vi "CFTS-Parse Data Header.vi"(8 "error in (no error)":errorcluster, 10 "Header string":string, 11 "Cluster Ref In":refnum<vi>) -> (0 "error out":errorcluster, 3 "Cluster Ref Out":refnum<vi>)   [LabVIEW 2020]
uses:
  <vilib>/regexp/Match Regular Expression.xnode
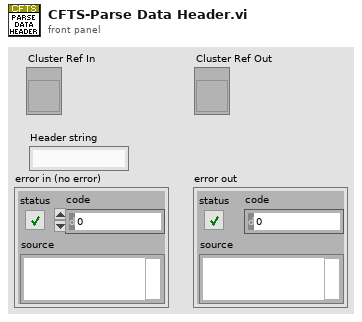
[diagram p1: front panel]
types:
  T1 = typedef "VariantType.lvlib/Type.ctl" = enum8{"Invalid Type", "Void", "I8", "I16", "I32", "I64", "U8", "U16", "U32", "U64", "Single Float", "Double Float", "Extended Float", "Single Complex", "Double Complex", "Extended Complex", "Enum U8", "Enum U16", "Enum U32", "Enum U64", "Single Float With Unit", "Double Float With Unit", "Extended Float With Unit", "Single Complex with Unit", "Double Complex with Unit", "Extended Complex with Unit", "Boolean", "String", "Path", "Picture", "Tag", "Array", "Cluster", "Variant", "LV Variant", "Waveform", "Timestamp", "Digital Waveform", "Digital Data", "ExpressData", "Refnum", "External Data", "VI", "Poly VI", "LabVIEW Class Instance", "Fixed Point"}
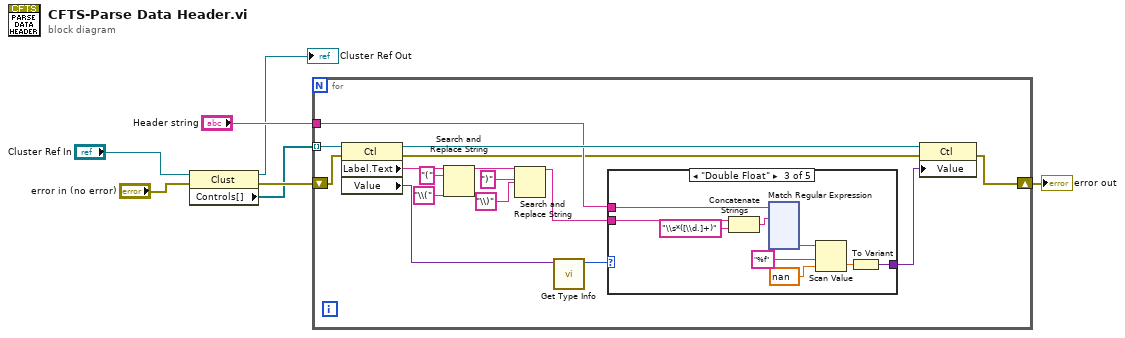
[diagram p0: block diagram]
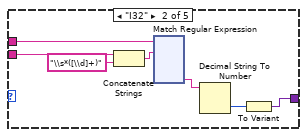
[diagram p3: hidden frame]
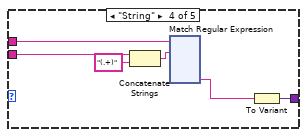
[diagram p4: hidden frame]
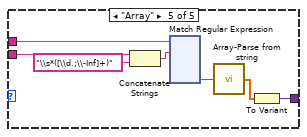
[diagram p5: hidden frame]
diagram:
  n1 = property class="Clust"(reference="Cluster Ref In", error in="error in (no error)") -> (reference out=→"Cluster Ref Out":refnum<vi>, error out=w7:errorcluster, "Controls[]"=w6:refnum<vi>[])
  n2 = for {
    tunnel: w6 -> [w23] mode=indexing
    tunnel: "Header string" -> [w18]
    shift-right: [w8] -> w3
    shift-left: w7 -> [w10]
    n3 = property class="Ctl"(reference=w23, error in=w10) -> (reference out=w20:refnum<vi>, error out=w9:errorcluster, "Label.Text"=w17:string, "Value"=w22:variant)
    n4 = Search and Replace String(input string=w17, search string="(", replace string="\\(" ("replace string (\"\")")) -> (result string=w14:string)  [unwired: 5 in, 3 out]
    n5 = Search and Replace String(input string=w14, search string=")", replace string="\\)" ("replace string (\"\")")) -> (result string=w13:string)  [unwired: 5 in, 3 out]
    n6 = call "Get Type Info.vi"("Variant"=w22) -> ("Type Enum"=w21:T1)  [unwired: 8 in, 2 out]
    n7 = case shown="\"Double Float\"" w21 {
      tunnel: [_ w30 w152 w271 w391] -> w19
      tunnel: w13 -> [_ w27 w149 w268 w388]
      tunnel: w18 -> [_ w28 w150 w269 w389]
      frame "Invalid Type", Default {
      }
      frame "I32" {
        n8 = Concatenate Strings(w27, "\\s*([\\d]+)" ("string")) -> (w29:string)
        n9 = xnode "Match Regular Expression"("input string"=w28, "regular expression"=w29) -> ("submatch 1"=w24:string)  [unwired: 4 in, 5 out]
        n10 = Decimal String To Number(string=w24) -> (number=w25:i32)  [unwired: 2 in, 1 out]
        n11 = To Variant(anything=w25) -> (Variant=w30:variant)
      }
      frame "Double Float" {
        n12 = Concatenate Strings(w149, "\\s*([\\d.]+)" ("string")) -> (w151:string)
        n13 = xnode "Match Regular Expression"("input string"=w150, "regular expression"=w151) -> ("submatch 1"=w146:string)  [unwired: 4 in, 5 out]
        n14 = Scan Value(string=w146, format string="%f", default (0 dbl)=nan) -> (value=w145:dbl)  [unwired: 1 out]
        n15 = To Variant(anything=w145) -> (Variant=w152:variant)
      }
      frame "String" {
        n16 = Concatenate Strings(w268, "(.+)" ("string")) -> (w270:string)
        n17 = xnode "Match Regular Expression"("input string"=w269, "regular expression"=w270) -> ("submatch 1"=w266:string)  [unwired: 4 in, 5 out]
        n18 = To Variant(anything=w266) -> (Variant=w271:variant)
      }
      frame "Array" {
        n19 = Concatenate Strings(w388, "\\s*([\\d.;\\-Inf]+)" ("string")) -> (w390:string)
        n20 = xnode "Match Regular Expression"("input string"=w389, "regular expression"=w390) -> ("submatch 1"=w386:string)  [unwired: 4 in, 5 out]
        n21 = call "Array-Parse from string.vi"("String"=w386) -> ("Array"=w385:dbl[])  [unwired: 13 in, 1 out]
        n22 = To Variant(anything=w385) -> (Variant=w391:variant)
      }
    }
    n23 = property class="Ctl"(reference=w20, error in=w9, "Value"=w19) -> (error out=w8:errorcluster)  [unwired: 1 out]
  }
  "error out" <- w3
